vi "VerifyData.vi"(5 "Data Size":i32, 7 "Index":i32, 8 "Data Buffer":u8[](array[numeric]) format="%.0x") -> (2 "Found":bool)   [LabVIEW 2010]
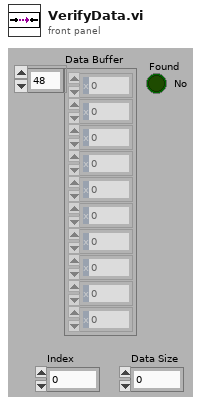
[diagram p1: front panel]
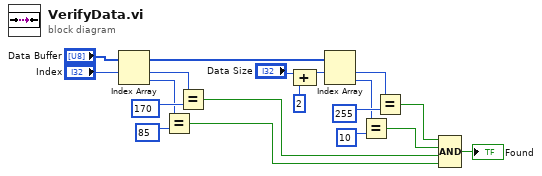
[diagram p0: block diagram]
diagram:
  n1 = Index Array(array="Data Buffer", index #1="Index") -> (element #1=w17:u8, element #2=w10:u8)  [unwired: 1 in]
  n2 = Equal?(x=w10, y=u8 85) -> (x = y?=w2:bool)
  n3 = Equal?(x=w17, y=u8 170) -> (x = y?=w3:bool)
  n4 = Compound Arithmetic op=ADD("Data Size", 2 ("value")) -> (w11:i32)
  n5 = Index Array(array="Data Buffer", index #1=w11) -> (element #1=w6:u8, element #2=w7:u8)  [unwired: 1 in]
  n6 = Equal?(x=w7, y=u8 10) -> (x = y?=w4:bool)
  n7 = Equal?(x=w6, y=u8 255) -> (x = y?=w5:bool)
  n8 = Compound Arithmetic op=AND(w5, w4, w3, w2) -> (→"Found":bool)
